vi "Update Console.vi"(6 "MessageType":T1, 7 "Message ID":u16, 9 "Message":string, 10 "Topic Name":string, 11 "Console In":string) -> (2 "Message String":string, 3 "Console Out":string)   [LabVIEW 2018]
uses:
  mqtt/Controls/MessageType.ctl
  mqtt/MQTT_Functions.lvlib
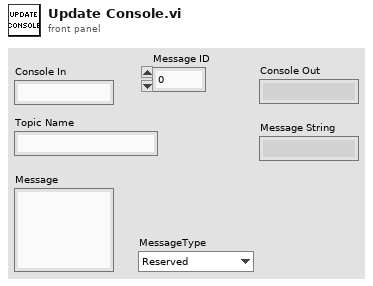
[diagram p1: front panel]
types:
  T1 = typedef "MQTT_Functions.lvlib/MessageType.ctl" = enum32{"Reserved", "CONNECT", "CONNACK", "PUBLISH", "PUBACK", "PUBREC", "PUBREL", "PUBCOMP", "SUBSCRIBE", "SUBACK", "UNSUBSCRIBE", "UNSUBACK", "PINGREQ", "PINGRESP", "DISCONNECT", "Reserved2"}
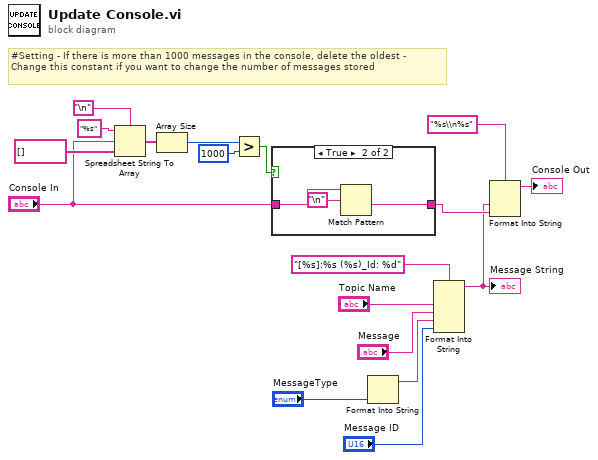
[diagram p0: block diagram]
diagram:
  # "#Setting - If there is more than 1000 messages in the console, delete the oldest - Change this constant if you want to change the number of messages stored"
  n1 = Spreadsheet String To Array(delimiter (Tab)="\n", format string="%s", spreadsheet string="Console In", array type (2D Dbl)=string[] []) -> (array=w8:string[])
  n2 = Array Size(array=w8) -> (size(s)=w3:i32)
  n3 = Greater?(x=w3, y=1000) -> (0:w5:bool)
  n4 = case shown="True" w5 {
    tunnel: [w19 w20] -> w2
    tunnel: "Console In" -> [w19 w21]
    frame False {
    }
    frame True {
      n5 = Match Pattern(string=w21, regular expression="\n") -> (after substring=w20:string)  [unwired: 1 in, 3 out]
    }
  }
  n6 = Format Into String("MessageType") -> (resulting string=w12:string)  [unwired: 3 in, 1 out]
  n7 = Format Into String(format string="[%s]:%s (%s)_Id: %d", "Topic Name", "Message", w12, "Message ID") -> (resulting string=w1:string)  [unwired: 2 in, 1 out]
  "Message String" <- w1
  n8 = Format Into String(format string="%s\\n%s", w1, w2) -> (resulting string=→"Console Out":string)  [unwired: 2 in, 1 out]
